vi "Preview Control States.vi"(8 "error in":errorcluster, 11 "Control in":refnum<class "Control.lvclass">) -> (0 "error out":errorcluster, 2 "States preview":picture[](array[picture]), 3 "Control out":refnum<class "Control.lvclass">)   [LabVIEW 2012, in "Control.lvclass"]
doc: "Get a preview (2D picture array) of the different expected button states."
uses:
  Control.lvclass
  Control.lvclass/Control.ctl
  <userlib>/BitMan/BitMap class/BitMap.lvclass
  <userlib>/BitMan/Built-in Filters class/Built-in Filters.lvclass
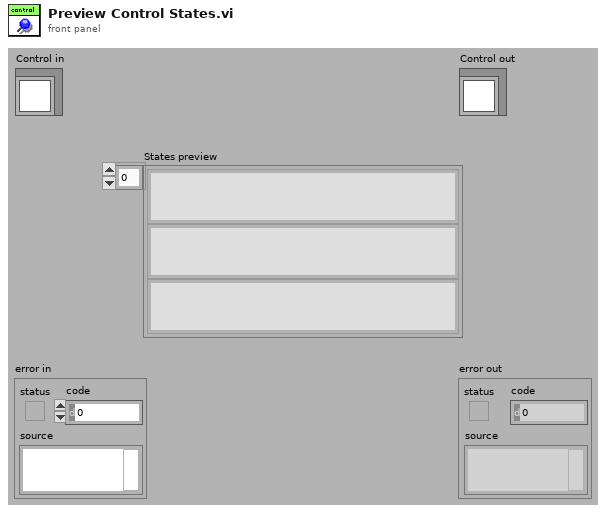
[diagram p1: front panel]
types:
  T1 = enum16{"User-specified Font", "Application Font", "System Font", "Dialog Font"}
  T2 = typedef "Control.lvclass/BX.Orientation__LCR _Modified.ctl" = u8
  T3 = typedef "Control.lvclass/_ui_tools_font.ctl" = cluster{"Font Name:":string, "Size":i16, "Strikeout?":bool, "Italic?":bool, "Underline?":bool, "Outline?":bool, "Shadow?":bool, "Bold?":bool}
  T4 = typedef "imagedata.ctl" = cluster{"image type":i32, "image depth":i32, "image":u8[], "mask":u8[], "colors":u32[], "Rectangle":cluster{"left":i16, "top":i16, "right":i16, "bottom":i16}}
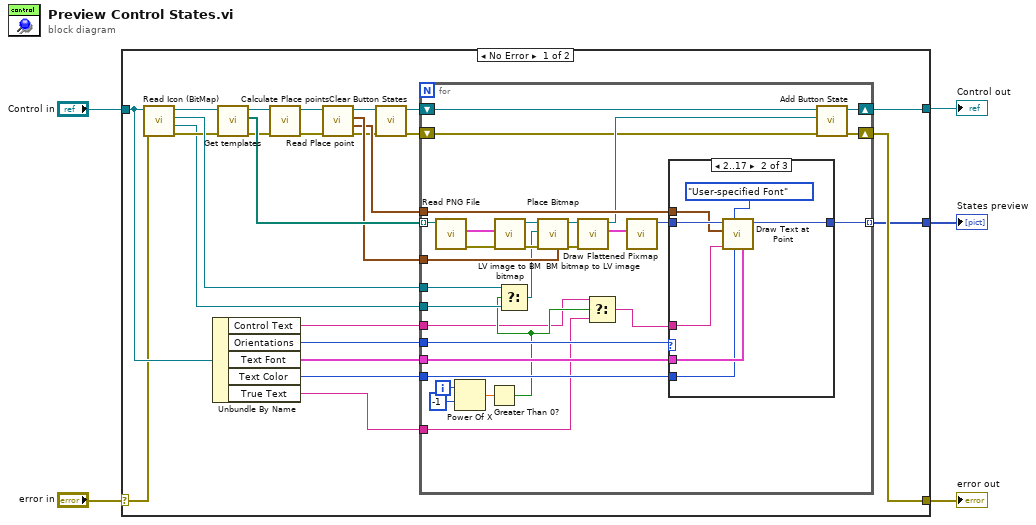
[diagram p0: block diagram]
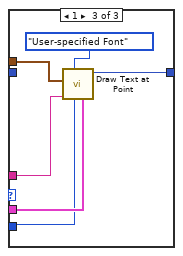
[diagram p3: hidden frame]
diagram:
  n1 = case shown="No Error" "error in" {
    selector: "error in" -> [w15 w76]
    tunnel: [w22 w76] -> w4
    tunnel: [w23 w75] -> w2
    tunnel: "Control in" -> [w19 w75]
    tunnel: [w21 _] -> w1
    frame No Error {
      n2 = call-dynamic "Read Icon (BitMap).vi"("error in (no error)"=w15, "Control in"=w19) -> ("error out"=w16:errorcluster, "Icon (BitMap) True"=w7:refnum<class "BitMap.lvclass">, "Icon (BitMap) False"=w27:refnum<class "BitMap.lvclass">, "Control out"=w17:refnum<class "Control.lvclass">)  [unwired: 6 out]
      n3 = Unbundle By Name(w19) -> ("Control Text"=w18:string, "Orientations"=w20:T2, "Text Font"=w10:T3, "Text Color"=w8:u32, "True Text"=w6:string)
      n4 = call-dynamic "Get templates.vi"("error in (no error)"=w16, "Control in"=w17) -> ("error out"=w14:errorcluster, "PNG templates"=w30:path[], "Control out"=w9:refnum<class "Control.lvclass">)  [unwired: 7 out]
      n5 = call-dynamic "Calculate Place points.vi"("error in (no error)"=w14, "Control in"=w9) -> ("error out"=w13:errorcluster, "Control out"=w28:refnum<class "Control.lvclass">)  [unwired: 8 out]
      n6 = call-dynamic "Read Place point.vi"("error in (no error)"=w13, "Control in"=w28) -> ("error out"=w11:errorcluster, "Text Point"=w26:cluster{"x":i32, "y":i32}, "Point"=w29:cluster{"x":i32, "y":i32}, "Control out"=w12:refnum<class "Control.lvclass">)  [unwired: 6 out]
      n7 = call-dynamic "Clear Button States.vi"("error in (no error)"=w11, "Control in"=w12) -> ("error out"=w24:errorcluster, "Control out"=w25:refnum<class "Control.lvclass">)  [unwired: 8 out]
      n8 = for {
        tunnel: w30 -> [w55] mode=indexing
        tunnel: [w50] -> w21 mode=indexing
        tunnel: w29 -> [w54]
        tunnel: w27 -> [w39]
        tunnel: w18 -> [w32]
        tunnel: w26 -> [w49]
        shift-right: [w47] -> w23
        shift-left: w25 -> [w48]
        shift-right: [w45] -> w22
        shift-left: w24 -> [w44]
        tunnel: w20 -> [w43]
        tunnel: w10 -> [w42]
        tunnel: w8 -> [w41]
        tunnel: w7 -> [w40]
        tunnel: w6 -> [w33]
        i -> [w37]
        n9 = call <vilib>:"Read PNG File.vi"("path to PNG file"=w55) -> ("error out"=w60:errorcluster, "image data"=w59:T4)  [unwired: 1 in, 8 out]
        n10 = Power Of X(1:-1 ("x"), 2:w37) -> (0:w35:dbl)
        n11 = Greater Than 0?(x=w35) -> (x > 0?=w34:bool)
        n12 = call <userlib>:"LV image to BM bitmap.vi"("error in (no error)"=w60, "LV image data"=w59) -> ("error out"=w52:errorcluster, "BitMap out"=w53:refnum<class "BitMap.lvclass">)  [unwired: 2 in, 6 out]
        n13 = Select(t=w39, s=w34, f=w40) -> (s? t:f=w38:refnum<class "BitMap.lvclass">)
        n14 = call <userlib>:"Place Bitmap.vi"("Place point"=w54, "error in (no error)"=w52, "Bitmap to place"=w38, "Bitmap in (optional)"=w53) -> ("error out"=w56:errorcluster, "Bitmap out"=w58:refnum<class "BitMap.lvclass">)  [unwired: 2 in, 4 out]
        n15 = call <userlib>:"BM bitmap to LV image.vi"("error in (no error)"=w56, "BitMap in"=w58) -> ("LV image data"=w57:T4, "BitMap out"=w46:refnum<class "BitMap.lvclass">)  [unwired: 1 in, 7 out]
        n16 = Select(t=w32, s=w34, f=w33) -> (s? t:f=w31:string)
        n17 = call <vilib>:"Draw Flattened Pixmap.vi"("image data"=w57) -> ("new picture"=w51:picture)  [unwired: 1 in, 7 out]
        n18 = case shown="2..17" w43 {
          tunnel: w31 -> [_ w68 w74]
          tunnel: w51 -> [w61 w67 _]
          tunnel: [w61 w66 w73] -> w50
          tunnel: w49 -> [_ w64 w71]
          tunnel: w42 -> [_ w63 w70]
          tunnel: w41 -> [_ w62 w69]
          frame Default {
          }
          frame 2..17 {
            n19 = call <vilib>:"Draw Text at Point.vi"("[user-specified font]"=w63, "text color(black)"=w62, "desired font(Application)"=T1."User-specified Font", "text"=w68, "origin"=w64, "picture"=w67) -> ("new picture"=w66:picture)  [unwired: 3 in, 2 out]
          }
          frame 1 {
            n20 = call <vilib>:"Draw Text at Point.vi"("[user-specified font]"=w70, "text color(black)"=w69, "desired font(Application)"=T1."User-specified Font", "text"=w74, "origin"=w71) -> ("new picture"=w73:picture)  [unwired: 4 in, 2 out]
          }
        }
        n21 = call-dynamic "Add Button State.vi"("error in (no error)"=w44, "State"=w46, "Control in"=w48) -> ("error out"=w45:errorcluster, "Control out"=w47:refnum<class "Control.lvclass">)  [unwired: 7 out]
      }
    }
    frame Error {
    }
  }
  "error out" <- w4
  "Control out" <- w2
  "States preview" <- w1
